vi "Read lifter config.vi"(0 "Insert name":enum16{"Insert #1", "Insert #2", "CALIB_INSERT"}(ring), 2 "File Name":string="Lifter config", 3 "Default":bool, 5 "error in (no error)":errorcluster) -> (6 "Lifter locations array":dbl[](array[numeric]), 8 "error out":errorcluster)   [LabVIEW 2019]
uses:
  <vilib>/Utility/config.llb/Read Key (Double).vi
  <vilib>/Utility/config.llb/NI_LVConfig.lvlib
panel:
  out "Top Cup possition":dbl
  out "middle cup possition":dbl
  out "bot possition":dbl
  out "appended path":path
  out "concatenated string":string
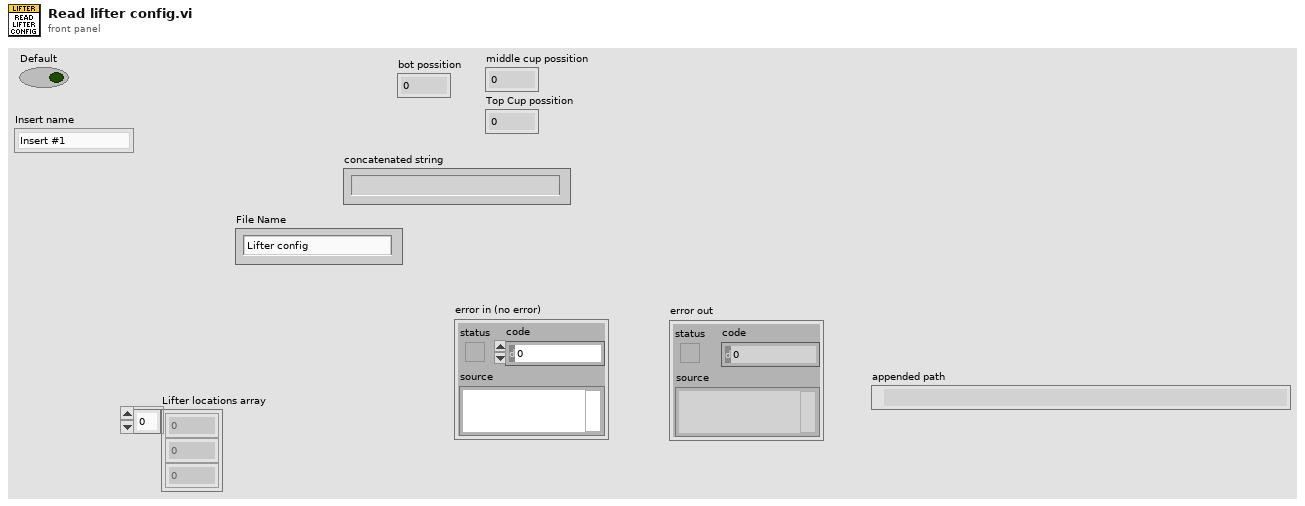
[diagram p1: front panel]
types:
  T1 = typedef "NI_LVConfig.lvlib/Config Data RefNum.ctl" = refnum<k1>
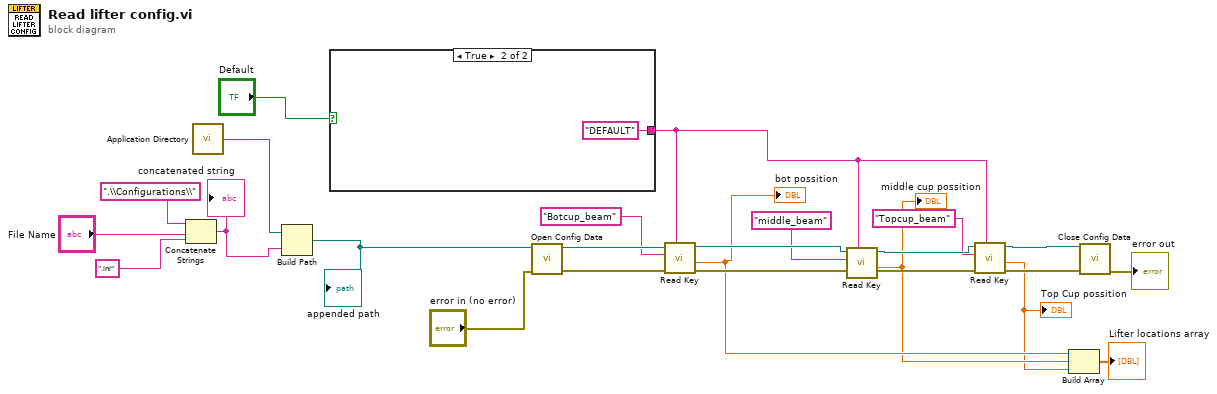
[diagram p0: block diagram]
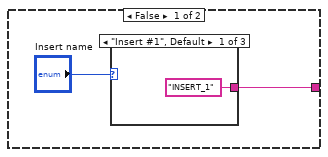
[diagram p2: hidden frame]
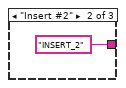
[diagram p3: hidden frame]
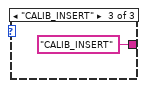
[diagram p4: hidden frame]
diagram:
  n1 = Concatenate Strings(".\\Configurations\\" ("string"), "File Name", ".ini" ("string")) -> (w22:string)
  "concatenated string" <- w22
  n2 = call <vilib>:"Application Directory.vi"() -> ("Application Directory"=w20:path)
  n3 = Build Path(base path=w20, name or relative path=w22) -> (appended path=w17:path)
  "appended path" <- w17
  n4 = case shown="True" "Default" {
    tunnel: [w25 "DEFAULT" ("section")] -> w2
    frame False {
      n5 = case shown="\"Insert #1\", Default" "Insert name" {
        tunnel: ["INSERT_1" ("section") "INSERT_2" ("section") "CALIB_INSERT" ("section")] -> w25
        frame "Insert #1", Default {
        }
        frame "Insert #2" {
        }
        frame "CALIB_INSERT" {
        }
      }
    }
    frame True {
    }
  }
  n6 = call <vilib>:"Open Config Data.vi"("error in (no error)"="error in (no error)", "configuration file path"=w17) -> ("error out"=w15:errorcluster, "refnum"=w16:T1)  [unwired: 7 in, 1 out]
  n7 = call-poly <vilib>:"Read Key.vi"("section"=w2, "error in (no error)"=w15, "key"="Botcup_beam" ("section"), "refnum"=w16) -> ("error out"=w10:errorcluster, "value"=w7:dbl, "refnum out"=w14:T1)  [unwired: 4 in, 1 out]
  "bot possition" <- w7
  n8 = call-poly <vilib>:"Read Key.vi"("section"=w2, "key"="middle_beam" ("section"), "refnum"=w14) -> ("value"=w6:dbl, "refnum out"=w13:T1)  [unwired: 5 in, 2 out]
  "middle cup possition" <- w6
  n9 = call-poly <vilib>:"Read Key.vi"("section"=w2, "error in (no error)"=w10, "key"="Topcup_beam" ("section"), "refnum"=w13) -> ("error out"=w11:errorcluster, "value"=w5:dbl, "refnum out"=w12:T1)  [unwired: 4 in, 1 out]
  "Top Cup possition" <- w5
  n10 = Build Array(w7, w6, w5) -> (→"Lifter locations array":dbl[])
  n11 = call <vilib>:"Close Config Data.vi"("error in (no error)"=w11, "refnum"=w12) -> ("error out"=→"error out":errorcluster)  [unwired: 8 in, 1 out]
